vi "测试-命令行调用python程序.vi"() -> ()   [LabVIEW 2018]
panel:
  out "字符串":string="未完成"
  out "布尔":bool
  out "standard output":string caption="标准输出"
  out "x+1":i32
  out "标尺.范围:最大值":dbl
  in  "关闭界面":bool
  out "模型预测进度（请等待）":u8(slide) scale=0.0..120.0
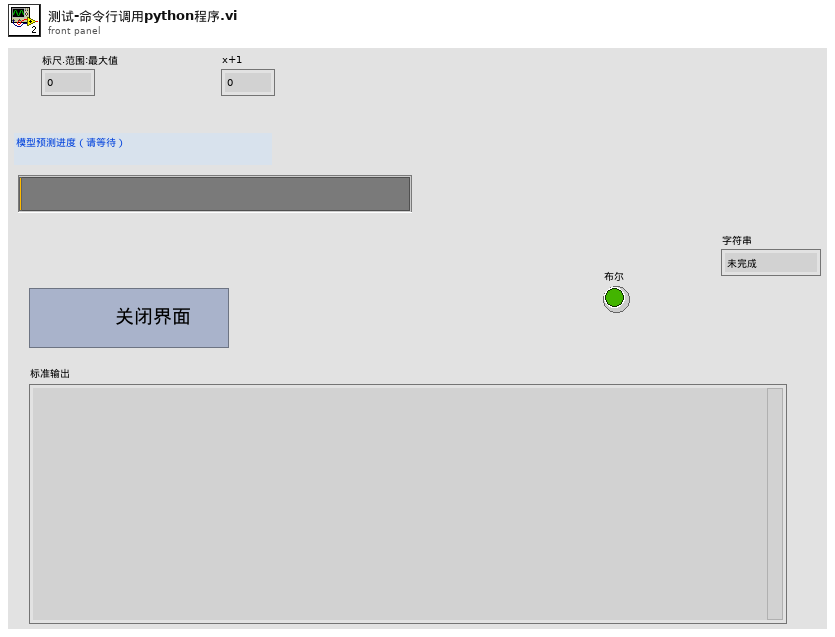
[diagram p1: front panel]
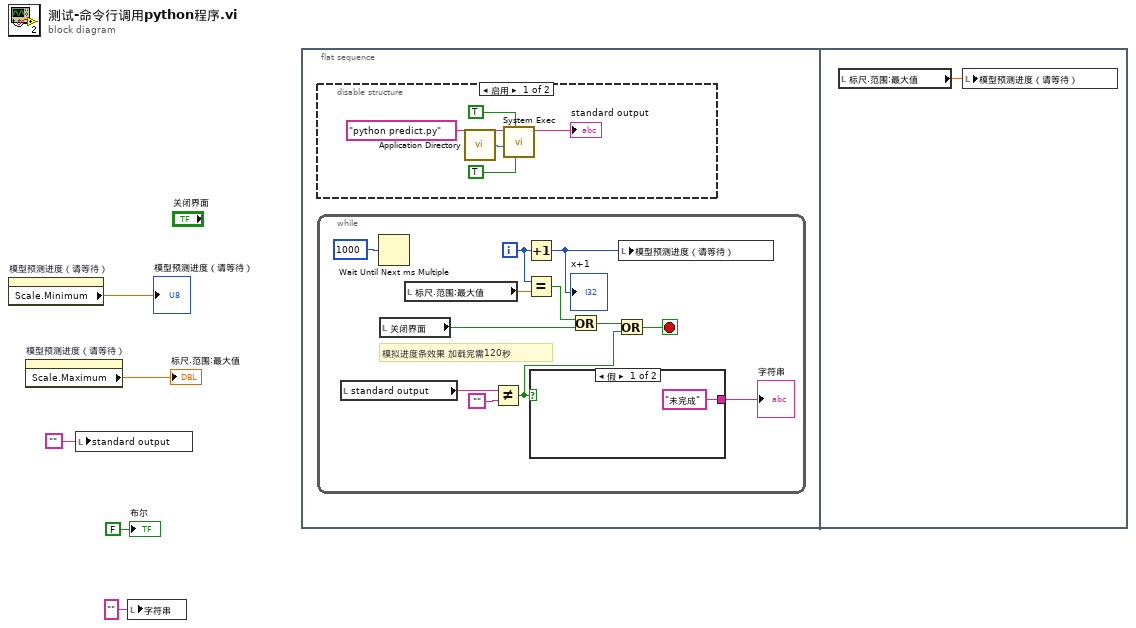
[diagram p0: block diagram]
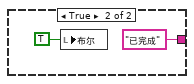
[diagram p3: hidden frame]
diagram:
  n1 = property on="模型预测进度（请等待）" class="Slide (严格)"() -> ("Scale.Minimum"=→"模型预测进度（请等待）":dbl)  [unwired: 2 in, 2 out]
  n2 = property on="模型预测进度（请等待）" class="Slide (严格)"() -> ("Scale.Maximum"=→"标尺.范围:最大值":dbl)  [unwired: 2 in, 2 out]
  n3 = local write "standard output"("") -> ()
  n4 = local write "字符串"("" ("字符串")) -> ()
  n5 = flat-sequence {
    frame #0 {
      n6 = disable-structure shown="启用" {
        frame Enabled {
          n7 = call <vilib>:"Application Directory.vi"() -> ("Application Directory"=w7:path)
          n8 = call <vilib>:"System Exec.vi"("run minimized? (F)"=TRUE, "wait until completion? (T)"=TRUE, "working directory"=w7, "command line"="python predict.py") -> ("standard output"=→"standard output":string)  [unwired: 4 in, 3 out]
        }
        frame Disabled {
        }
      }
      n9 = while {
        i -> [w20]
        stop <- w13 stop-if-true
        # "模拟进度条效果 加载完需120秒"
        n10 = local read "standard output"() -> (w16:string)
        n11 = Wait Until Next ms Multiple(millisecond multiple=u32 1000 ("毫秒倍数")) -> ()  [unwired: 1 out]
        n12 = local read "关闭界面"() -> (w19:bool)
        n13 = local read "标尺.范围:最大值"() -> (w17:dbl)
        n14 = Not Equal?(x=w16, y="") -> (x != y?=w12:bool)
        n15 = Increment(x=w20) -> (x+1=w21:i32)
        "x+1" <- w21
        n16 = Equal?(x=w20, y=w17) -> (x = y?=w18:bool)
        n17 = case shown="假" w12 {
          tunnel: ["未完成" "已完成"] -> w11
          frame False {
          }
          frame True {
            n18 = local write "布尔"(TRUE ("布尔")) -> ()
          }
        }
        "字符串" <- w11
        n19 = Or(x=w18, y=w19) -> (x .or. y?=w14:bool)
        n20 = Or(x=w14, y=w12) -> (x .or. y?=w13:bool)
        n21 = local write "模型预测进度（请等待）"(w21) -> ()
      }
    }
    frame #1 {
      n22 = local read "标尺.范围:最大值"() -> (w26:dbl)
      n23 = local write "模型预测进度（请等待）"(w26) -> ()
    }
  }
  "布尔" <- FALSE ("布尔")
